vi "Convert Pass-Fail to String.vi"(11 "Pass?":bool) -> (3 "Pass/Fail String":string)   [LabVIEW 2020, in "MacroAssert.lvlib"]
doc: "Converts <B>Pass?</B> to a pass/fail string to be displayed."
uses:
  MacroAssert.lvlib
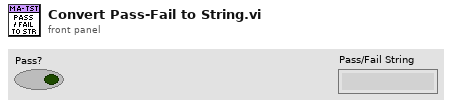
[diagram p1: front panel]
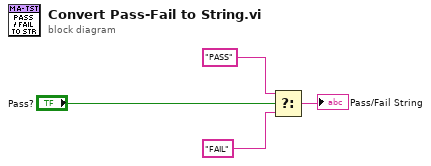
[diagram p0: block diagram]
diagram:
  n1 = Select(t="PASS", s="Pass?", f="FAIL") -> (s? t:f=→"Pass/Fail String":string)
